vi "oa_Speed Profile Property String Constant.vi"() -> (4 "pulse/rev":string="NI_OA_Pulse_Per_Rev", 6 "speed profile":string="NI_OA_Speed_Profile", 10 "elapsed time":string="NI_OA_ELapsed_Time", 15 "rotation direction":string="NI_OA_Rotation_Direction")   [LabVIEW 2017]
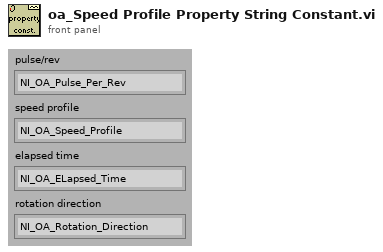
[diagram p1: front panel]
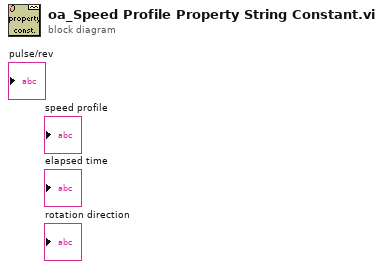
[diagram p0: block diagram]
diagram:
